vi "lautstärkeregelung.vi"(0 "Referenz":refnum<vi>, 1 "Referenz 2":refnum<vi>, 2 "Referenz 3":refnum<vi>, 3 "musik lautstärke optionen":T1(radio) caption="Titel-volume-options", 4 "Volume":i64(slide) min=0 max=100 scale=0.1..100.0) -> (5 "volume out":dbl)   [LabVIEW 2010]
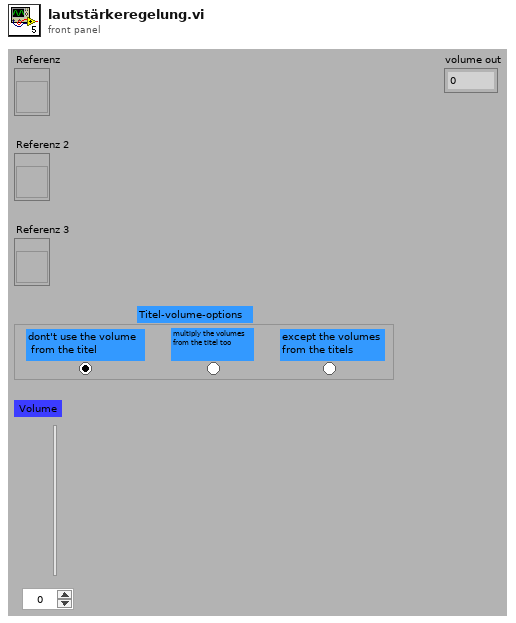
[diagram p1: front panel]
types:
  T1 = enum32{"ohne", "dazu", "von der Playlist übernehmen"}
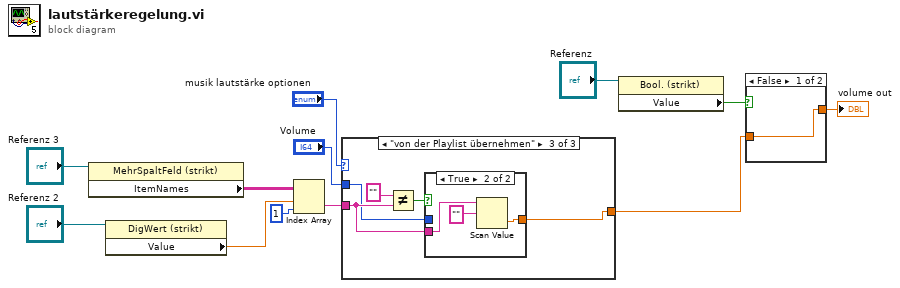
[diagram p0: block diagram]
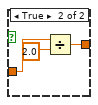
[diagram p2: hidden frame]
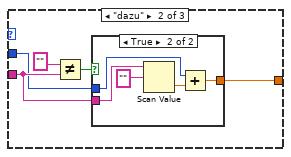
[diagram p4: hidden frame]
diagram:
  n1 = property on="Eigenschaftsknoten" class="MehrSpaltFeld (strikt)"(reference="Referenz 3") -> ("ItemNames"=w12:string[][])  [unwired: 1 in, 2 out]
  n2 = property class="DigWert (strikt)"(reference="Referenz 2") -> ("Value"=w6:dbl)  [unwired: 1 in, 2 out]
  n3 = Index Array(array=w12, index (row)=w6, index (col)=1 ("Deaktivierter Index (Spalte)")) -> (element=w4:string)
  n4 = case shown="\"von der Playlist übernehmen\"" "musik lautstärke optionen" {
    tunnel: w4 -> [_ w16 w27]
    tunnel: "Volume" -> [w13 w15 w25]
    tunnel: [w13 w14 w26] -> w10
    frame "ohne", Default {
    }
    frame "dazu" {
      n5 = Not Equal?(x="", y=w16) -> (x != y?=w17:bool)
      n6 = case shown="TRUE" w17 {
        tunnel: w16 -> [_ w22]
        tunnel: w15 -> [w19 w24]
        tunnel: [w19 w23] -> w14
        frame False {
        }
        frame True {
          n7 = Scan Value(string=w22, format string="" ("Format-String")) -> (value=w21:dbl)  [unwired: 2 out]
          n8 = Add(x=w24, y=w21) -> (x+y=w23:dbl)
        }
      }
    }
    frame "von der Playlist übernehmen" {
      n9 = Not Equal?(x="", y=w27) -> (x != y?=w28:bool)
      n10 = case shown="TRUE" w28 {
        tunnel: w27 -> [_ w33]
        tunnel: [w30 w32] -> w26
        tunnel: w25 -> [w30 _]
        frame False {
        }
        frame True {
          n11 = Scan Value(string=w33, format string="" ("Format-String")) -> (value=w32:dbl)  [unwired: 2 out]
        }
      }
    }
  }
  n12 = property class="Bool. (strikt)"(reference="Referenz") -> ("Value"=w9:bool)  [unwired: 1 in, 2 out]
  n13 = case shown="FALSE" w9 {
    tunnel: w10 -> [w34 w37]
    tunnel: [w34 w35] -> w11
    frame False {
    }
    frame True {
      n14 = Divide(x=w37, y=2.0) -> (x/y=w35:dbl)
    }
  }
  "volume out" <- w11
